vi "ParameterUI.vi"() -> ()   [LabVIEW 2013, in "Parameter.lvclass"]
doc: "Template for creating new user-interface VIs for inherited classes."
uses:
  Parameter.lvclass
  <vilib>/NI/AMC/Message Queue.ctl
  <vilib>/NI/AMC/Message.ctl
  <vilib>/NI/Tools/Keyed Array/KeyedArray.ctl
  xCE/xceTreeObj/xceTreeObj.lvclass
  channel_dataType.ctl
  Parameter.lvclass/Parameter.ctl
  <vilib>/NI/AMC/Read Termination Message.vi
  <vilib>/NI/AMC/Create Single Message.vi
  <vilib>/NI/AMC/Update Message Routing Info.vi
  <vilib>/NI/AMC/Send Message.vi
  <vilib>/NI/AMC/Globals.vi
  <vilib>/NI/AMC/AMC.lvlib
  xCE/xceDataNode/xceDataNode.lvclass
  <vilib>/NI/Tools/Keyed Array/Tools_KeyedArray.lvlib
panel:
  in  "Data Type":T1=enum."U32"
  in  "Offset":dbl format="%#.6g"
  in  "Scale":dbl format="%#.6g"
  in  "Initial Value":dbl format="%#.6g"
  in  "Name":string
  in  "Control Name":string
  in  "DataNode*":refnum<data-value>
  in  "AMC*":T2
  in  "Exit":bool
  # "The Name of the Control in the FPGA VI"
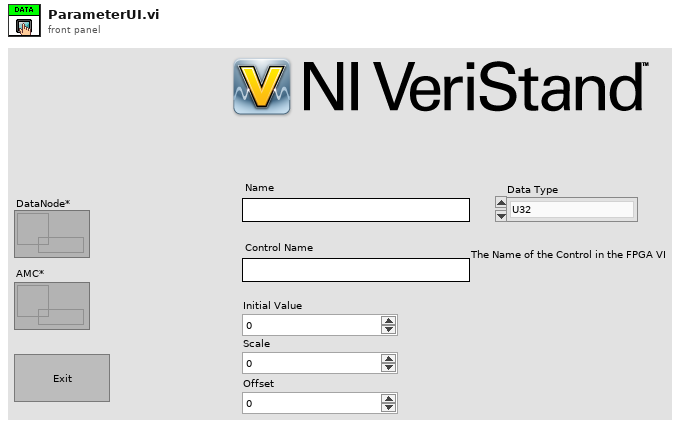
[diagram p1: front panel]
types:
  T1 = typedef "Parameter.lvclass/channel_dataType.ctl" = enum16{"Boolean", "U8", "I8", "U16", "I16", "U32", "I32", "U64", "I64", "FXPI32", "FXPU32", "FXPI64", "FXPU64", "PWM"}
  T2 = typedef "AMC.lvlib/Message Queue.ctl" = refnum<queue>
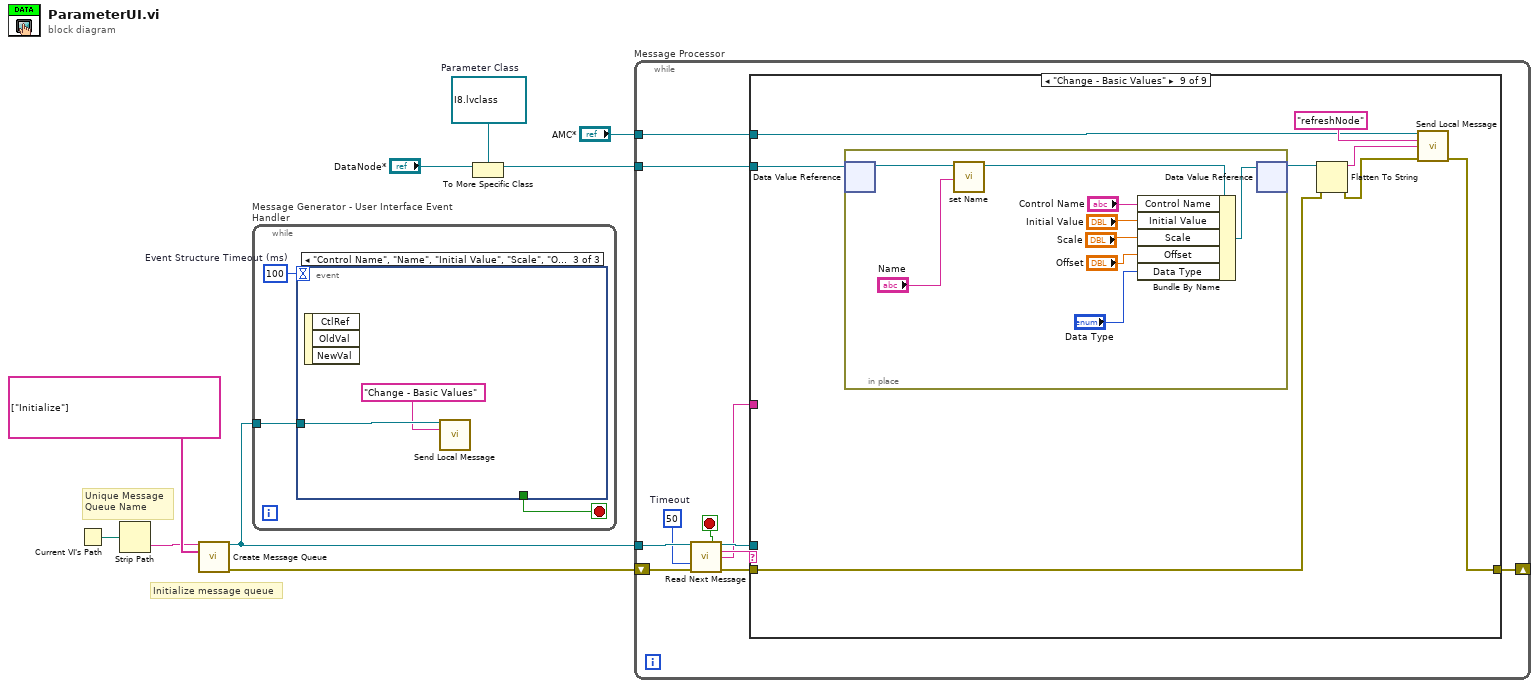
[diagram p0: block diagram]
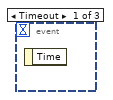
[diagram p2: hidden frame]
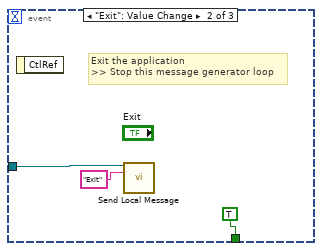
[diagram p3: hidden frame]
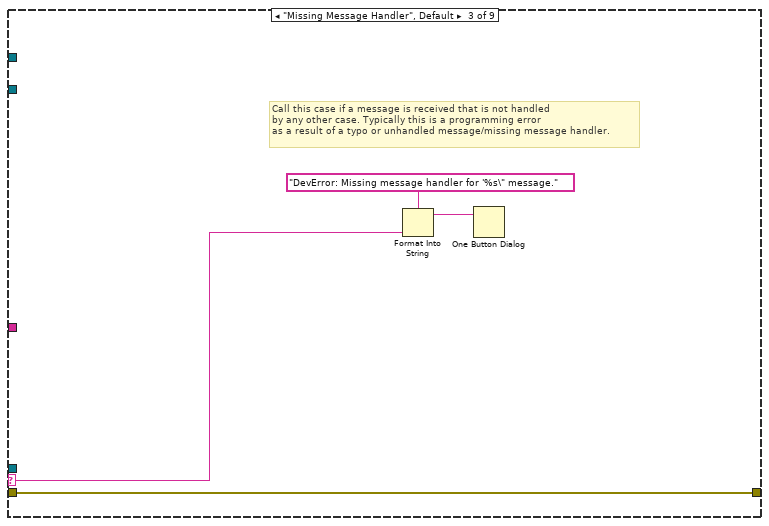
[diagram p6: hidden frame]
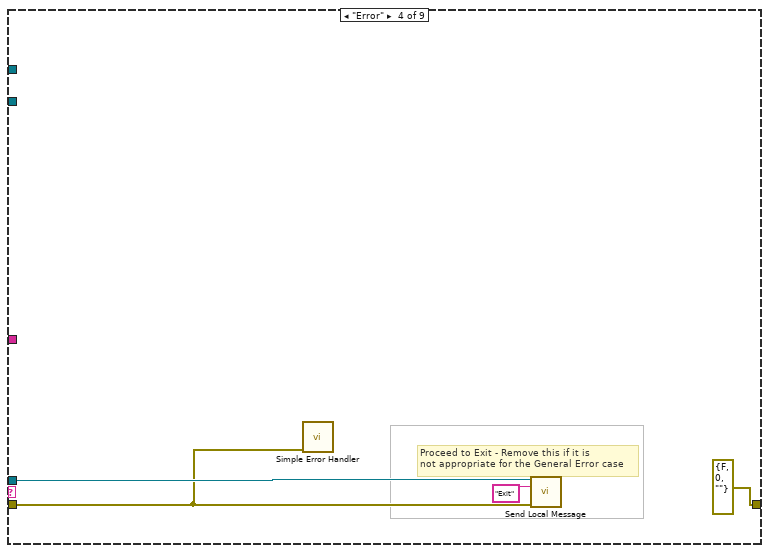
[diagram p7: hidden frame]
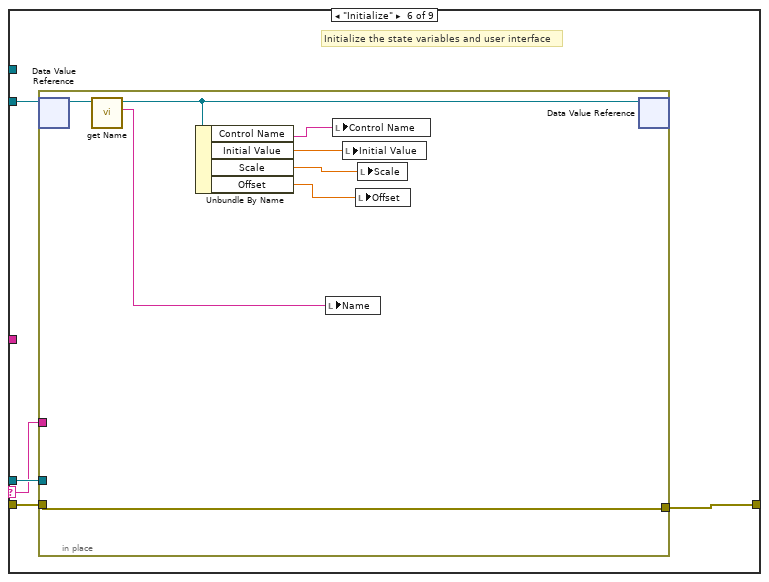
[diagram p9: hidden frame]
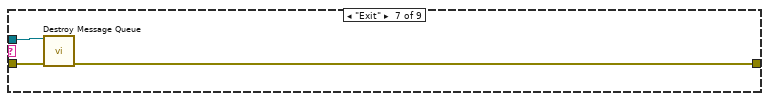
[diagram p10: hidden frame]
diagram:
  w1 = refnum<data-value> refnum  # Parameter Class
  # "Initialize message queue"
  # "Unique Message\nQueue Name"
  n1 = Current VI's Path() -> (path=w5:path)
  n2 = Strip Path(path=w5) -> (name=w8:string)  [unwired: 1 out]
  n3 = call <vilib>:"Create Message Queue.vi"("message queue name"=w8, "initial message names"=string[] ["Initialize"]) -> ("message queue out"=w7:T2, "error out"=w6:errorcluster)  [unwired: 12 in]
  n4 = while "Message Generator - User Interface Event Handler" {
    tunnel: w7 -> [w10]
    stop <- w11 stop-if-true
    w12 = 100  # Event Structure Timeout (ms)
    n5 = event shown="[2] \"Control Name\", \"Name\", \"Initial Value\", \"Scale\", \"Offset\": Value Change" {
      selector: _ -> [_ _ _]
      dyn-events: _ -> [_ _ _]
      timeout: w12 -> [_ _ _]
      tunnel: [_ TRUE ("Discard?") _] -> w11
      tunnel: w10 -> [_ w13 w17]
      event Timeout {
        n6 = event-data() -> ()  [unwired: 2 out]
      }
      event "Exit": Value Change {
        # "Exit the application\n>> Stop this message generator loop"
        n7 = event-data() -> ()  [unwired: 2 out]
        n8 = call <vilib>:"Send Local Message.vi"("message queue in"=w13, "message name"="Exit") -> ()  [unwired: 11 in, 3 out]
      }
      event "Control Name", "Name", "Initial Value", "Scale", "Offset": Value Change {
        n9 = event-data() -> ()  [unwired: 4 out]
        n10 = call <vilib>:"Send Local Message.vi"("message queue in"=w17, "message name"="Change - Basic Values" ("Message Name")) -> ()  [unwired: 11 in, 3 out]
      }
    }
  }
  n11 = To More Specific Class(target class=w1, reference="DataNode*") -> (specific class reference=w2:refnum<data-value>)  [unwired: 1 in, 1 out]
  n12 = while "Message Processor" {
    shift-left: w6 -> [w25]
    shift-right: [w18] -> _
    tunnel: w7 -> [w26]
    tunnel: "AMC*" -> [w19]
    tunnel: w2 -> [w20]
    stop <- w28 stop-if-true
    w23 = 50  # Timeout
    n13 = call <vilib>:"Read Next Message.vi"("message queue in"=w26, "timeout (1 ms)"=w23, "error in"=w25) -> ("exit process?"=w28:bool, "message queue out"=w27:T2, "message name"=w22:string, "message value"=w21:string, "error out"=w24:errorcluster)  [unwired: 5 in, 3 out]
    n14 = case shown="\"Change - Basic Values\"" w22 {
      selector: w22 -> [_ _ w34 _ _ w40 _ _ _]
      tunnel: w27 -> [_ _ _ w38 _ w42 w54 _ _]
      tunnel: w24 -> [w29 w30 w31 w36 w39 w43 w55 w56 w58]
      tunnel: w21 -> [_ _ _ _ _ _ _ _ _]
      tunnel: w20 -> [_ _ _ _ _ w44 _ _ w64]
      tunnel: w19 -> [_ _ _ _ _ _ _ _ w60]
      tunnel: [w29 w30 w31 errorcluster {"status"=FALSE, "code"=0, "source"=""} ("error out") w39 w41 w53 w56 w57] -> w18
      frame "---------- Framework Operations ----------" {
        # "Dummy case to add a seperator in the Case Structure menu"
      }
      frame "", "Idle" {
      }
      frame "Missing Message Handler", Default {
        # "Call this case if a message is received that is not handled \nby any other case. Typically this is a programming error\nas a result of a typo or unhandled message/missing message handler."
        n15 = Format Into String(format string="DevError: Missing message handler for '%s\" message." ("message"), w34) -> (resulting string=w32:string)  [unwired: 2 in, 1 out]
        n16 = One Button Dialog(message=w32) -> ()  [unwired: 2 out]
      }
      frame "Error" {
        # "Proceed to Exit - Remove this if it is\nnot appropriate for the General Error case"
        n17 = call <vilib>:"Simple Error Handler.vi"("error in (no error)"=w36) -> ()  [unwired: 1 in, 8 out]
        n18 = call <vilib>:"Send Local Message.vi"("message queue in"=w38, "message name"="Exit", "error in"=w36) -> ()  [unwired: 10 in, 3 out]
      }
      frame "---------- Generic Operations ----------" {
        # "Dummy case to add a seperator in the Case Structure menu"
      }
      frame "Initialize" {
        # "Initialize the state variables and user interface"
        n19 = in-place {
          in-place-border: w43 -> [w50]
          in-place-border: w42 -> [_]
          in-place-border: [w50] -> w41
          in-place-border: w40 -> [_]
          n20 = in-place-dvr #1(w44) -> (w51:refnum<class "Parameter.lvclass">)  [unwired: 1 out]
          n21 = call "get Name.vi"("xceDataNode in"=w51) -> ("Name"=w52:string, "xceDataNode out"=w49:refnum<class "Parameter.lvclass">)  [unwired: 8 in, 1 out]
          n22 = Unbundle By Name(w49) -> ("Control Name"=w47:string, "Initial Value"=w48:dbl, "Scale"=w46:dbl, "Offset"=w45:dbl)
          n23 = local write "Name"(w52) -> ()
          n24 = local write "Control Name"(w47) -> ()
          n25 = local write "Initial Value"(w48) -> ()
          n26 = local write "Offset"(w45) -> ()
          n27 = local write "Scale"(w46) -> ()
          n28 = in-place-dvr #1(w49) -> ()  [unwired: 2 out]
        }
      }
      frame "Exit" {
        n29 = call <vilib>:"Destroy Message Queue.vi"("message queue in"=w54, "error in"=w55) -> ("error out"=w53:errorcluster)  [unwired: 11 in, 2 out]
      }
      frame "---------- Application Operations ----------" {
        # "Dummy case to add a seperator in the Case Structure menu"
      }
      frame "Change - Basic Values" {
        n30 = in-place {
          n31 = in-place-dvr #2(w64) -> (w70:refnum<class "Parameter.lvclass">)  [unwired: 1 out]
          n32 = call "set Name.vi"("Name"="Name", "xceDataNode in"=w70) -> ("xceDataNode out"=w72:refnum<class "Parameter.lvclass">)  [unwired: 8 in, 1 out]
          n33 = Bundle By Name(cluster=w72, "Control Name"="Control Name", "Initial Value"="Initial Value", "Scale"="Scale", "Offset"="Offset", "Data Type"="Data Type") -> (w73:refnum<class "Parameter.lvclass">)
          n34 = in-place-dvr #2(w73) -> (w59:refnum<data-value>)  [unwired: 1 out]
        }
        n35 = Flatten To String(anything=w59, error in (no error)=w58) -> (data string=w63:string, error out=w61:errorcluster)  [unwired: 2 in, 1 out]
        n36 = call <vilib>:"Send Local Message.vi"("message queue in"=w60, "message name"="refreshNode" ("Message Name"), "message value"=w63, "error in"=w61) -> ("error out"=w57:errorcluster)  [unwired: 9 in, 2 out]
      }
    }
  }
